vi "Exercise 3.1 ADC PCF8591.vi"() -> ()   [LabVIEW 2014]
uses:
  <vilib>/Q-Wave Systems/QwaveSys RPi Training Package (Demo)/Addons/QwaveSys RPi Training Library.lvlib
panel:
  in  "DAC":u8(knob) scale=0.0..255.0
  out "A3-Loop Back with AO":i32(knob) scale=0.0..255.0
  out "A2-VR Ristor":i32(knob) scale=0.0..255.0
  out "A1-Light Sensor":i32(knob) scale=0.0..255.0
  out "A0-Thermister":i32(knob) scale=0.0..255.0
  out "error out":errorcluster
  in  "error in (no error)":errorcluster
  # "Connect the shorting cap P4 P4 , select thermistor access circuit\n  Connect the shorting cap P5 P5 , select photoresistor access circuit\n  Connect the shorting cap P6 P6 , select 0-5V Adjustable voltage access circuit"
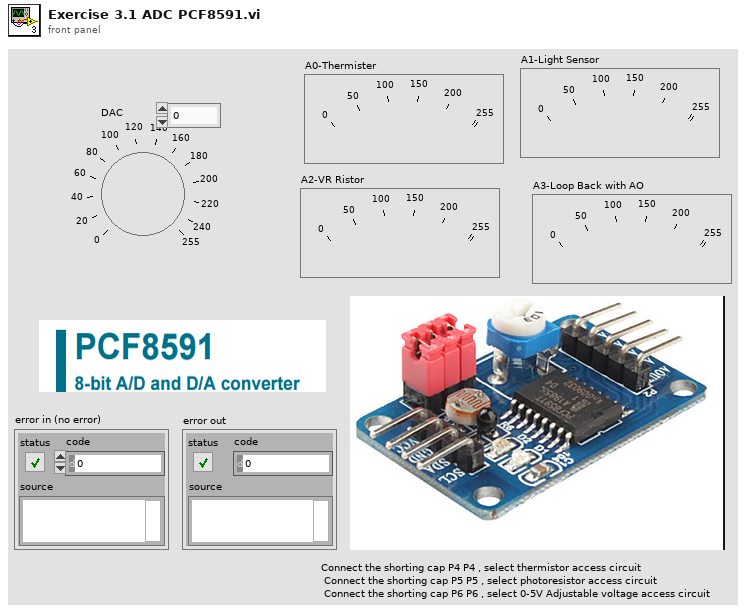
[diagram p1: front panel]
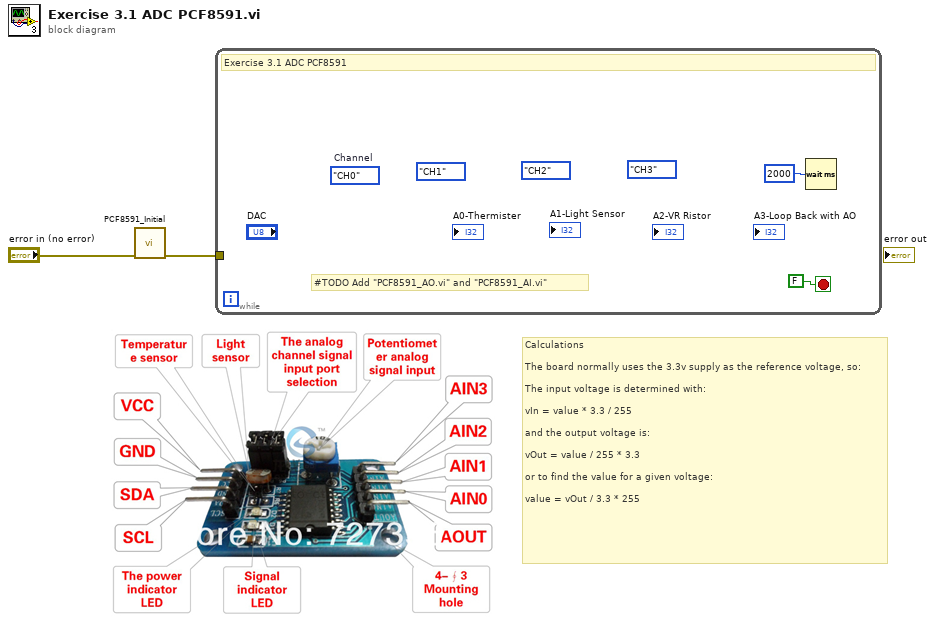
[diagram p0: block diagram]
diagram:
  # "Calculations\n\nThe board normally uses the 3.3v supply as the reference voltage, so:\n\nThe input voltage is determined with:\n\nvIn = value * 3.3 / 255\n\nand the output voltage is:\n\nvOut = value / 255 * 3.3\n\nor to find the value for a given voltage:\n\nvalue = vOut / 3.3 * 255"
  n1 = call <vilib>:"PCF8591_Initial.vi"("error in (no error)"="error in (no error)") -> ("error out"=w2:errorcluster)  [unwired: 10 in]
  n2 = while {
    tunnel: w2 -> [_]
    stop <- FALSE stop-if-true
    (unwired) enum16{"CH0", "CH1", "CH2", "CH3"}."CH3" ("Channel")
    (unwired) enum16{"CH0", "CH1", "CH2", "CH3"}."CH2" ("Channel")
    (unwired) enum16{"CH0", "CH1", "CH2", "CH3"}."CH1" ("Channel")
    (unwired) enum16{"CH0", "CH1", "CH2", "CH3"}."CH0"  # Channel
    # "#TODO Add \"PCF8591_AO.vi\" and \"PCF8591_AI.vi\""
    # "Exercise 3.1 ADC PCF8591"
    n3 = Wait (ms)(milliseconds to wait=u32 2000) -> ()  [unwired: 1 out]
  }
